vi "Create File.vi"(8 "error in":errorcluster) -> (0 "error out":errorcluster)   [LabVIEW 2018, in "Support Library.lvlib" / "Command Logging.lvlib"]
uses:
  Command Logging.lvlib
  <vilib>/Utility/sysdir.llb/System Directory Type.ctl
  File Path.ctl
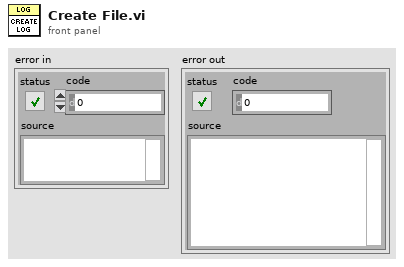
[diagram p1: front panel]
types:
  T1 = typedef "System Directory Type.ctl" = i32
  T2 = enum16{"open", "replace", "create", "open or create", "replace or create", "replace or create with confirmation"}
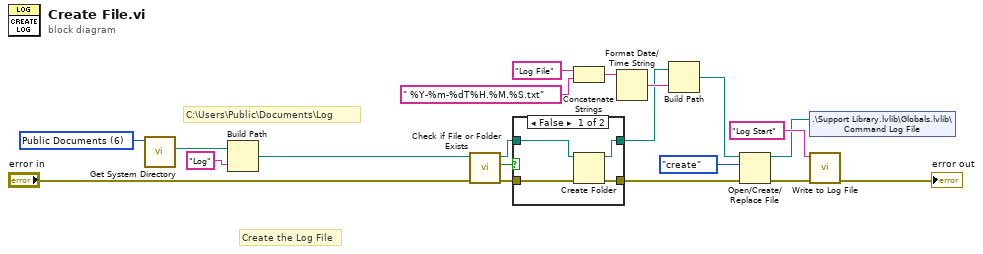
[diagram p0: block diagram]
diagram:
  w19 = T1 6 items=["User Home"=0, "User Desktop"=1, "User Documents"=2, "User Application Data"=3, "User Preferences"=4, "User Temporary"=5, "Public Documents"=6, "Public Application Data"=7, "Public Preferences"=8, "Public Cache"=13, "System Core Libraries"=9, "System Installed Libraries"=10, "Application Files"=11, "Boot Volume Root"=12] ("system directory type")
  # "Create the Log File"
  # "C:\\Users\\Public\\Documents\\Log"
  n1 = call <vilib>:"Get System Directory.vi"("system directory type"=w19) -> ("system directory"=w13:path)  [unwired: 10 in]
  n2 = Build Path(base path=w13, name or relative path="Log") -> (appended path=w4:path)
  n3 = call <vilib>:"Check if File or Folder Exists.vi"("error in (no error)"="error in", "path"=w4) -> ("error out"=w7:errorcluster, "file or folder exists?"=w6:bool, "dup path"=w5:path)  [unwired: 7 in]
  n4 = case shown="False" w6 {
    tunnel: w5 -> [w24 w26]
    tunnel: w7 -> [w23 w25]
    tunnel: [w22 w26] -> w3
    tunnel: [w21 w25] -> w1
    frame False {
      n5 = Create Folder(path (use dialog)=w24, error in=w23) -> (created path=w22:path, error out=w21:errorcluster)  [unwired: 1 in, 1 out]
    }
    frame True {
    }
  }
  n6 = Concatenate Strings("Log File" ("string"), " %Y-%m-%dT%H.%M.%S.txt" ("time format string (%c)")) -> (w14:string)
  n7 = Format Date/Time String(time format string (%c)=w14) -> (date/time string=w18:string)  [unwired: 2 in]
  n8 = Build Path(base path=w3, name or relative path=w18) -> (appended path=w15:path)
  n9 = Open/Create/Replace File(file path (use dialog)=w15, error in=w1, operation (0:open)=T2."create") -> (refnum out=w8:refnum<file>, error out=w11:errorcluster)  [unwired: 3 in, 1 out]
  n10 = shared-variable ".\\Support Library.lvlib\\Globals.lvlib\\Command Log File"(w8) -> ()  [unwired: 1 in, 1 out]
  n11 = call "Write to Log File.vi"("error in"=w11, "text"="Log Start") -> ("error out"=→"error out":errorcluster)  [unwired: 9 in]
